vi "Arm Control.vi"(5 "kd":dbl, 7 "kp":dbl, 9 "Current Speed":dbl, 10 "Current Height":dbl, 11 "Desired Height":dbl) -> (0 "In Range?":bool, 3 "Motor Output":dbl)   [LabVIEW 2014]
panel:
  in  "Range":dbl=0.2
  out "Graph":dbl(graph)
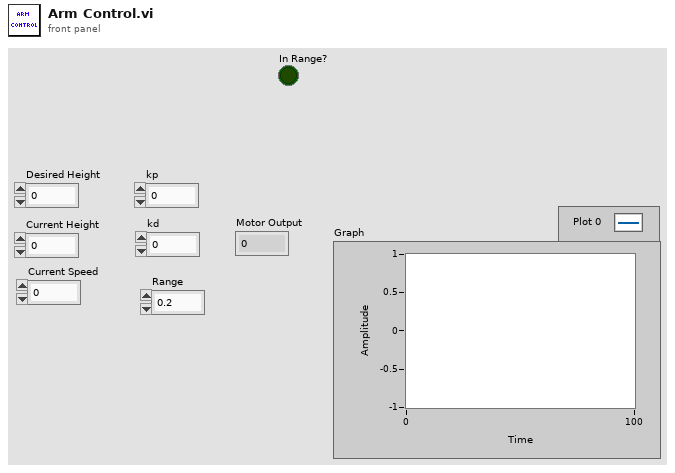
[diagram p1: front panel]
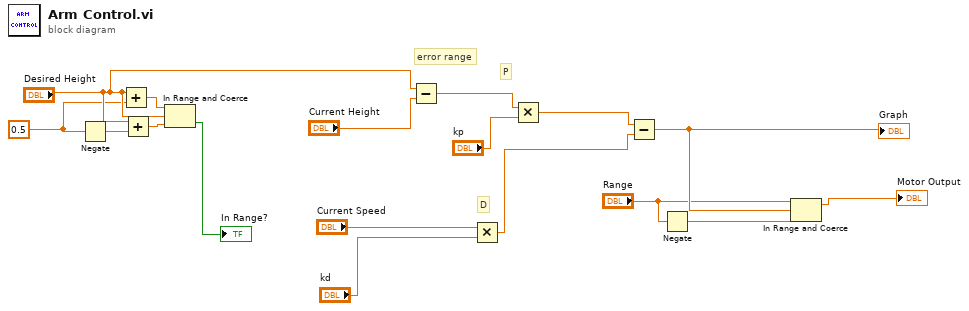
[diagram p0: block diagram]
diagram:
  w1 = 0.5
  # "D"
  # "P"
  # "error range"
  n1 = Negate(x=w1) -> (-x=w16:dbl)
  n2 = Add(x="Desired Height", y=w1) -> (x+y=w17:dbl)
  n3 = Add(x="Desired Height", y=w16) -> (x+y=w15:dbl)
  n4 = In Range and Coerce(upper limit=w17, x="Desired Height", lower limit=w15) -> (In Range?=→"In Range?":bool)  [unwired: 1 out]
  n5 = Subtract(x="Desired Height", y="Current Height") -> (x-y=w11:dbl)
  n6 = Multiply(x="Current Speed", y="kd") -> (x*y=w6:dbl)
  n7 = Multiply(x=w11, y="kp") -> (x*y=w7:dbl)
  n8 = Subtract(x=w7, y=w6) -> (x-y=w5:dbl)
  "Graph" <- w5
  n9 = Negate(x="Range") -> (-x=w3:dbl)
  n10 = In Range and Coerce(upper limit="Range", x=w5, lower limit=w3) -> (coerced(x)=→"Motor Output":dbl)  [unwired: 1 out]
